vi "OpenAppendFile.vi"(8 "error in (no error)":errorcluster caption="エラー入力（エラーなし）", 11 "ファイルパス（ダイアログを使用）":path) -> (0 "error out":errorcluster caption="エラー出力", 3 "refnum出力":refnum<file>)   [LabVIEW 2014]
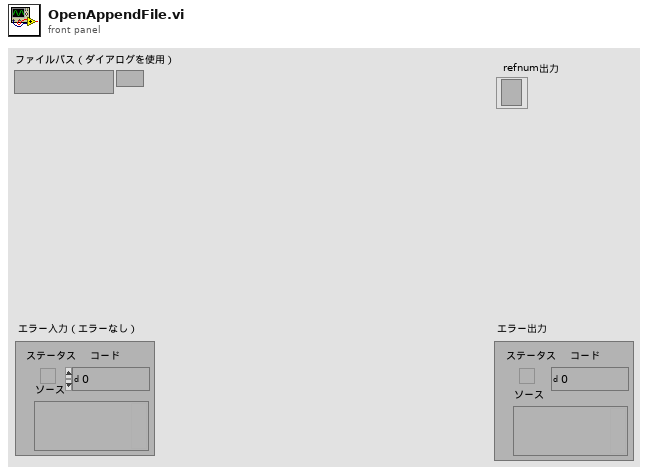
[diagram p1: front panel]
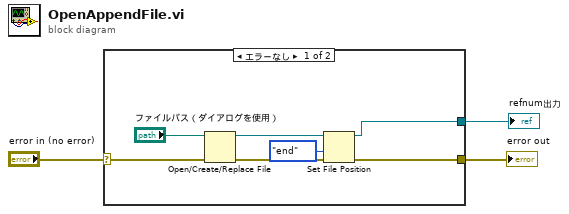
[diagram p0: block diagram]
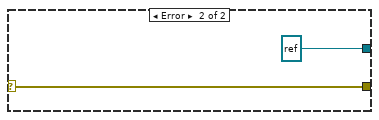
[diagram p2: hidden frame]
diagram:
  n1 = case shown="エラーなし" "error in (no error)" {
    selector: "error in (no error)" -> [w10 w12]
    tunnel: [w5 w12] -> w2
    tunnel: [w4 refnum<file> refnum ("refnum")] -> w1
    frame No Error {
      n2 = Open/Create/Replace File(file path (use dialog)="ファイルパス（ダイアログを使用）", error in=w10) -> (refnum out=w7:refnum<file>, error out=w6:errorcluster)  [unwired: 4 in, 1 out]
      n3 = Set File Position(refnum=w7, from (0:start)=enum16{"start", "end", "current"}."end" ("基点（0:start）"), error in=w6) -> (refnum out=w4:refnum<file>, error out=w5:errorcluster)  [unwired: 1 in]
    }
    frame Error {
    }
  }
  "error out" <- w2
  "refnum出力" <- w1
